vi "__getDaylightSavings.vi"() -> (0 "DST":i32)   [LabVIEW 2020]
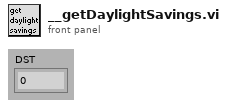
[diagram p1: front panel]
types:
  T1 = typedef "LVDateTimeRec.ctl" = cluster{"fractional second":dbl, "second":i32, "minute":i32, "hour":i32, "day of month":i32, "month":i32, "year":i32, "day of week":i32, "day of year":i32, "DST":i32}
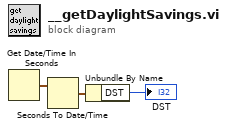
[diagram p0: block diagram]
diagram:
  n1 = Get Date/Time In Seconds() -> (seconds since 1Jan1904=w1:timestamp)
  n2 = Seconds To Date/Time(time stamp (now)=w1) -> (date time rec=w2:T1)  [unwired: 1 in]
  n3 = Unbundle By Name(w2) -> ("DST"=→"DST":i32)
